vi "Filter Byte Array.vi"(6 "Frame Read Init":bool, 8 "Total no of bytes":u16, 9 "EOH":u16, 10 "SOH":u16, 11 "Array Input":u16[](array[numeric])) -> (0 "Stop notifier":bool, 1 "Frame read":u32, 2 "Filtered array":u16[](array[numeric]), 3 "Second packet":u16[](array[numeric]), 4 "Second Packet notifier":bool)   [LabVIEW 2020]
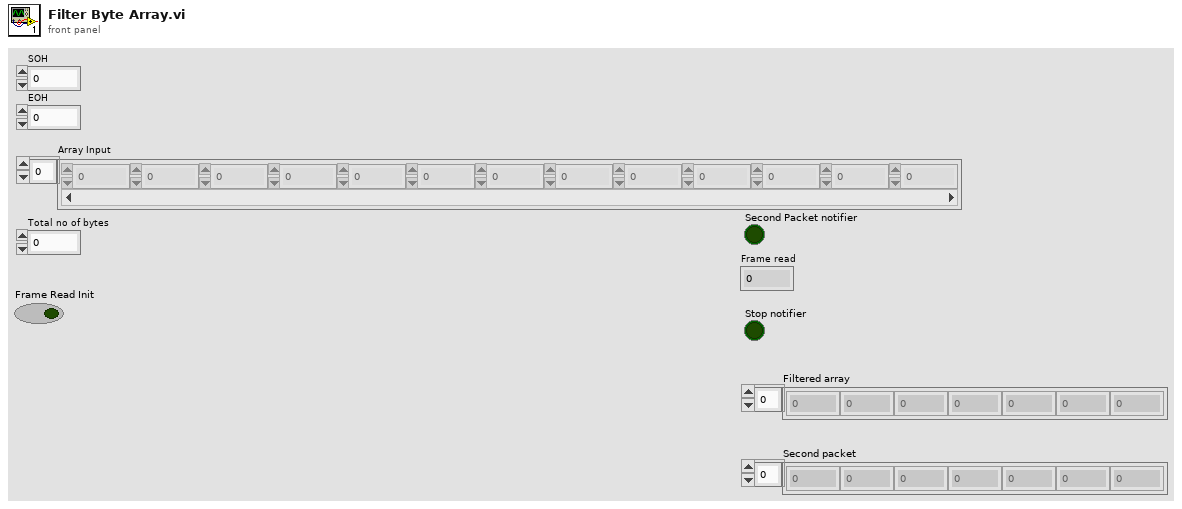
[diagram p1: front panel]
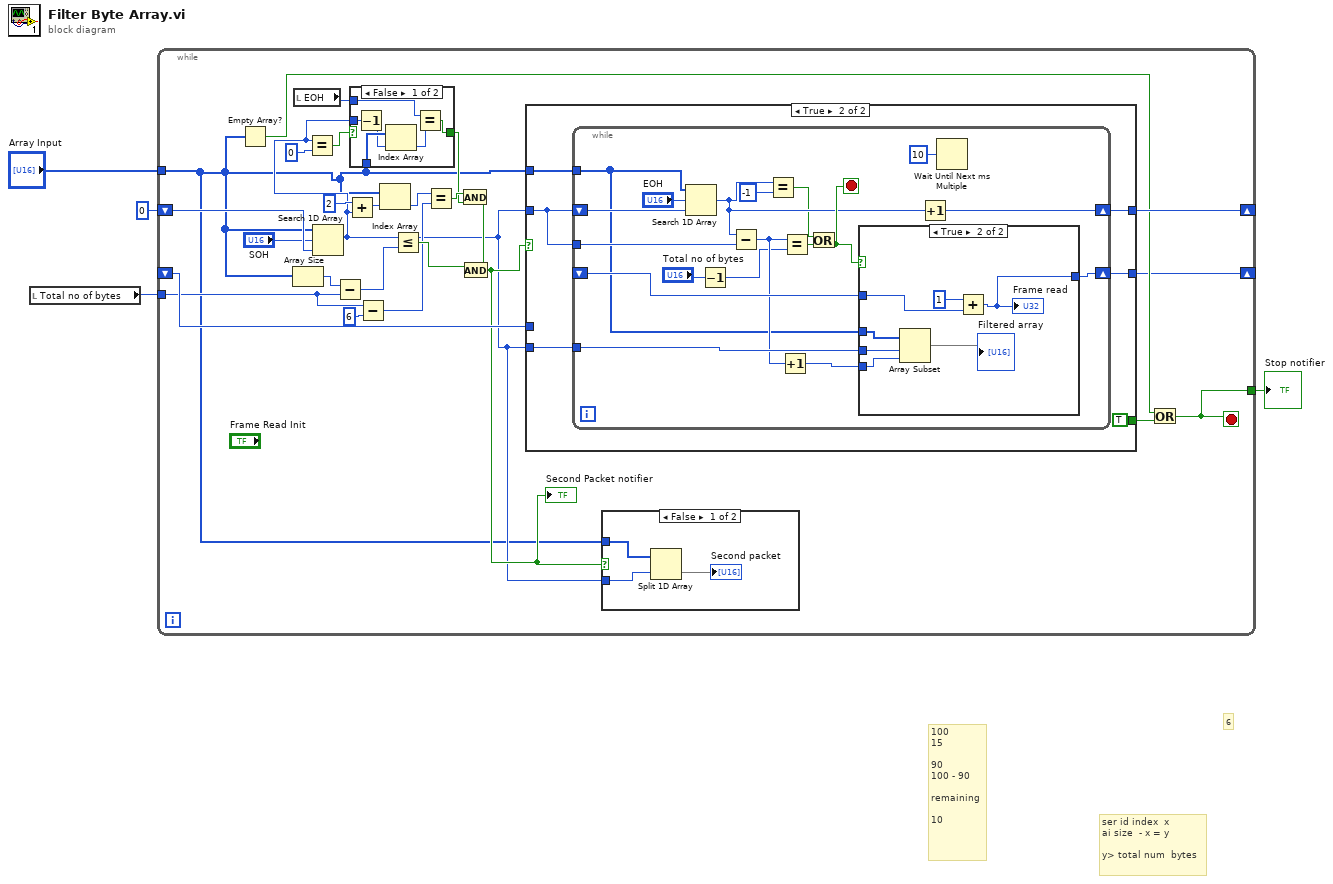
[diagram p0: block diagram]
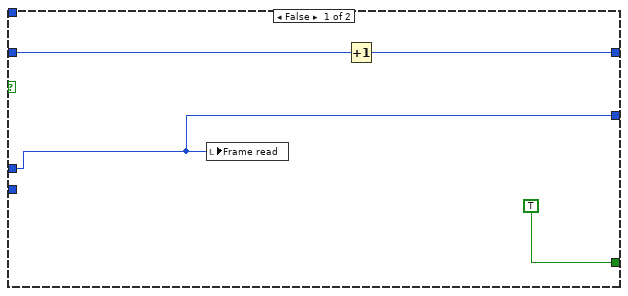
[diagram p4: hidden frame]
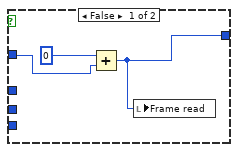
[diagram p5: hidden frame]
diagram:
  # "ser id index  x\nai size  - x = y\n\ny> total num  bytes"
  # "6"
  # "100\n15\n\n90\n100 - 90\n\nremaining\n\n10"
  n1 = local read "Total no of bytes"() -> (w3:u16)
  n2 = while {
    tunnel: "Array Input" -> [w7]
    shift-right: [w29] -> _
    shift-left: 0 ("index of element") -> [w30]
    shift-right: [w5] -> _
    shift-left: _ -> [w24]
    tunnel: w3 -> [w14]
    tunnel: [w22] -> w2
    stop <- w22 stop-if-true
    n3 = Empty Array?(array=w7) -> (empty?=w23:bool)
    n4 = Array Size(array=w7) -> (size(s)=w27:i32)
    n5 = local read "EOH"() -> (w6:u16)
    n6 = Search 1D Array(1D array=w7, element="SOH", start index (0)=w30) -> (index of element=w8:i32)
    n7 = Equal?(x=w8, y=0) -> (x = y?=w11:bool)
    n8 = Subtract(x=w27, y=w14) -> (x-y=w26:i32)
    n9 = Add(x=2, y=w8) -> (x+y=w20:i32)
    n10 = case shown="False" w11 {
      selector: w11 -> [_ w37]
      tunnel: [w31 w37] -> w9
      tunnel: w8 -> [w35 _]
      tunnel: w7 -> [w36 _]
      tunnel: w6 -> [w32 _]
      frame False {
        n11 = Decrement(x=w35) -> (x-1=w34:i32)
        n12 = Index Array(array=w36, index=w34) -> (element=w33:u16)
        n13 = Equal?(x=w32, y=w33) -> (x = y?=w31:bool)
      }
      frame True {
      }
    }
    n14 = Subtract(x=w14, y=u16 6) -> (x-y=w15:u16)
    n15 = Index Array(array=w7, index=w20) -> (element=w18:u16)
    n16 = Less Or Equal?(x=w8, y=w26) -> (x <= y?=w21:bool)
    n17 = Equal?(x=w18, y=w15) -> (x = y?=w17:bool)
    n18 = And(x=w17, y=w9) -> (x .and. y?=w10:bool)
    n19 = And(x=w21, y=w10) -> (x .and. y?=w16:bool)
    "Second Packet notifier" <- w16
    n20 = case shown="True" w16 {
      tunnel: [w41 w47] -> w29
      tunnel: w7 -> [_ w50]
      tunnel: w8 -> [w44 w49]
      tunnel: [TRUE TRUE] -> w25
      tunnel: w24 -> [w42 _]
      tunnel: w8 -> [_ w48]
      tunnel: [w42 w46] -> w5
      frame False {
        n21 = local write "Frame read"(w42) -> ()
        n22 = Increment(x=w44) -> (x+1=w41:i32)
      }
      frame True {
        n23 = while {
          tunnel: w50 -> [w58]
          shift-right: [w56] -> w47
          shift-left: w49 -> [w68]
          tunnel: w49 -> [w67]
          shift-right: [w64] -> w46
          shift-left: _ -> [w65]
          tunnel: w48 -> [w62]
          stop <- w55 stop-if-true
          n24 = Search 1D Array(1D array=w58, element="EOH", start index (0)=w68) -> (index of element=w54:i32)
          n25 = Decrement(x="Total no of bytes") -> (x-1=w57:u16)
          n26 = Subtract(x=w54, y=w67) -> (x-y=w61:i32)
          n27 = Equal?(x=w54, y=-1) -> (x = y?=w52:bool)
          n28 = Increment(x=w61) -> (x+1=w60:i32)
          n29 = Equal?(x=w61, y=w57) -> (x = y?=w59:bool)
          n30 = Or(x=w52, y=w59) -> (x .or. y?=w55:bool)
          n31 = case shown="True" w55 {
            tunnel: w65 -> [w70 w76]
            tunnel: [w69 w77] -> w64
            tunnel: w58 -> [_ w75]
            tunnel: w62 -> [_ w73]
            tunnel: w60 -> [_ w72]
            frame False {
              n32 = Add(x=u32 0, y=w70) -> (x+y=w69:u32)
              n33 = local write "Frame read"(w69) -> ()
            }
            frame True {
              n34 = Array Subset(array=w75, index=w73, length=w72) -> (→"Filtered array":u16[])
              n35 = Add(x=1, y=w76) -> (x+y=w77:u32)
              "Frame read" <- w77
            }
          }
          n36 = Increment(x=w54) -> (x+1=w56:i32)
          n37 = Wait Until Next ms Multiple(millisecond multiple=u32 10 ("milliseconds to wait")) -> ()  [unwired: 1 out]
        }
      }
    }
    n38 = case shown="False" w16 {
      tunnel: w7 -> [w40 _]
      tunnel: w8 -> [w39 _]
      frame False {
        n39 = Split 1D Array(array=w40, index=w39) -> (second subarray=→"Second packet":u16[])  [unwired: 1 out]
      }
      frame True {
      }
    }
    n40 = Or(x=w23, y=w25) -> (x .or. y?=w22:bool)
  }
  "Stop notifier" <- w2
